vi "zad4.vi"(8 "error in (no error)":errorcluster, 9 "Max":dbl, 10 "Min":dbl, 11 "N":dbl) -> (1 "error out":errorcluster, 2 "Array":dbl[](array[numeric]))   [LabVIEW 2017]
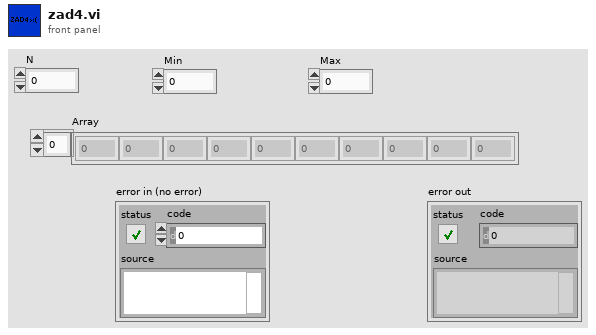
[diagram p1: front panel]
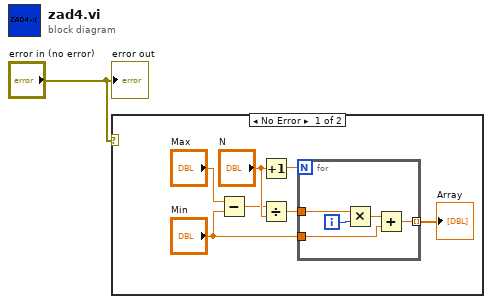
[diagram p0: block diagram]
diagram:
  n1 = case shown="No Error" "error in (no error)" {
    frame No Error {
      n2 = Subtract(x="Max", y="Min") -> (x-y=w5:dbl)
      n3 = Increment(x="N") -> (x+1=w7:dbl)
      n4 = Divide(x=w5, y="N") -> (x/y=w4:dbl)
      n5 = for {
        N: w7 -> [_]
        tunnel: w4 -> [w13]
        tunnel: "Min" -> [w10]
        tunnel: [w9] -> w2 mode=indexing
        i -> [w12]
        n6 = Multiply(x=w13, y=w12) -> (x*y=w11:dbl)
        n7 = Add(x=w11, y=w10) -> (x+y=w9:dbl)
      }
      "Array" <- w2
    }
    frame Error {
    }
  }
  "error out" <- "error in (no error)"
